vi "Subtract RF Hammer.vi"(3 "error in (no error)":errorcluster, 4 "RF Hammer Queue":refnum<queue>, 5 "Breakdown Signal":waveform(dbl)[](array[waveform])) -> (0 "error out":errorcluster, 1 "Average RF Hammer":waveform(dbl)[](array[waveform]), 2 "Reduced Signal":waveform(dbl)[](array[waveform]))   [LabVIEW 2013, in "Breakdown Acoustics Controls.lvlib"]
uses:
  Breakdown Acoustics Controls.lvlib
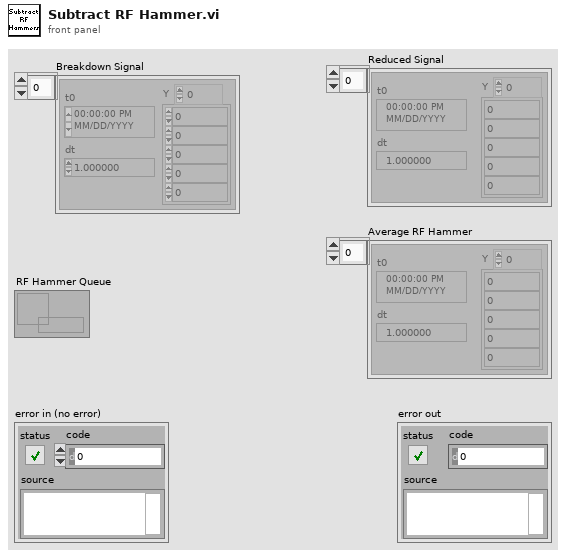
[diagram p1: front panel]
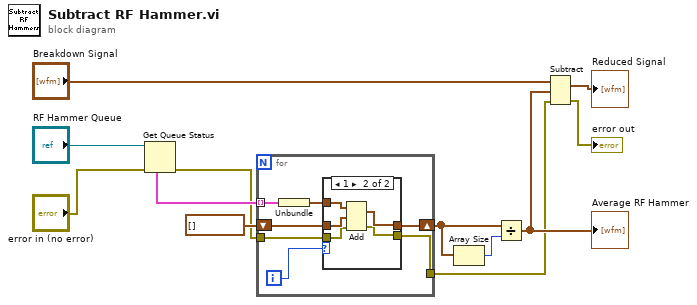
[diagram p0: block diagram]
diagram:
  n1 = Get Queue Status(queue="RF Hammer Queue", error in (no error)="error in (no error)") -> (error out=w6:errorcluster, elements=w10:cluster{waveform(dbl)[]}[])  [unwired: 1 in, 6 out]
  n2 = for {
    tunnel: w10 -> [w17] mode=indexing
    shift-right: [w18] -> w7
    shift-left: waveform(dbl)[] [] -> [w15]
    tunnel: w6 -> [w14]
    tunnel: [w13] -> w2
    i -> [w19]
    n3 = Unbundle(w17) -> (w16:waveform(dbl)[])
    n4 = case shown="1" w19 {
      tunnel: w16 -> [w21 w25]
      tunnel: [w21 w24] -> w18
      tunnel: w15 -> [_ w26]
      tunnel: w14 -> [w20 w23]
      tunnel: [w20 w22] -> w13
      frame 0, Default {
      }
      frame 1 {
        n5 = Add(1:w26, 2:w25, 4:w23) -> (0:w24:waveform(dbl)[], 3:w22:errorcluster)
      }
    }
  }
  n6 = Array Size(array=w7) -> (size(s)=w8:i32)
  n7 = Divide(x=w7, y=w8) -> (x/y=w4:waveform(dbl)[])
  "Average RF Hammer" <- w4
  n8 = Subtract(1:w4, 2:"Breakdown Signal", 4:w2) -> (0:→"Reduced Signal":waveform(dbl)[], 3:→"error out":errorcluster)
